vi "generateModels_v1.vi"() -> ()   [LabVIEW 2019]
panel:
  in  "DEV scan no":string="0011"
  out "SCAN_NO":string
  out "PC Processed":bool
  out "ACh Processed":bool
  in  "Build Model":bool
  in  "Process VSCAN":bool
  in  "stop":bool
  # ">>>"
  # ">>>"
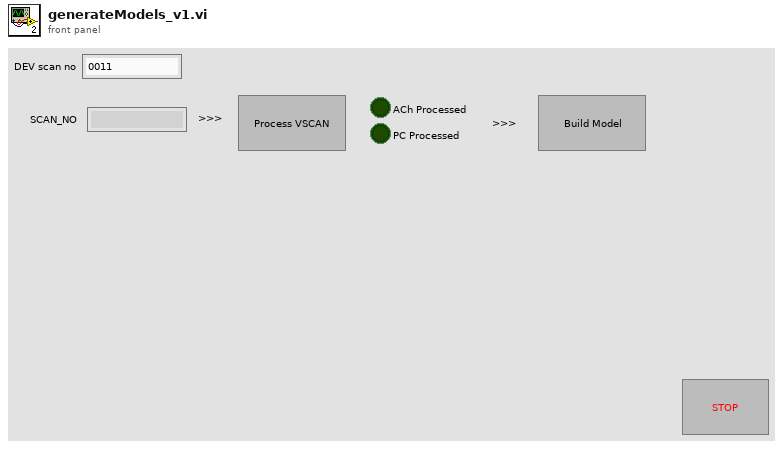
[diagram p1: front panel]
types:
  T1 = enum8{"Enabled", "Disabled", "Disabled and Grayed Out"}
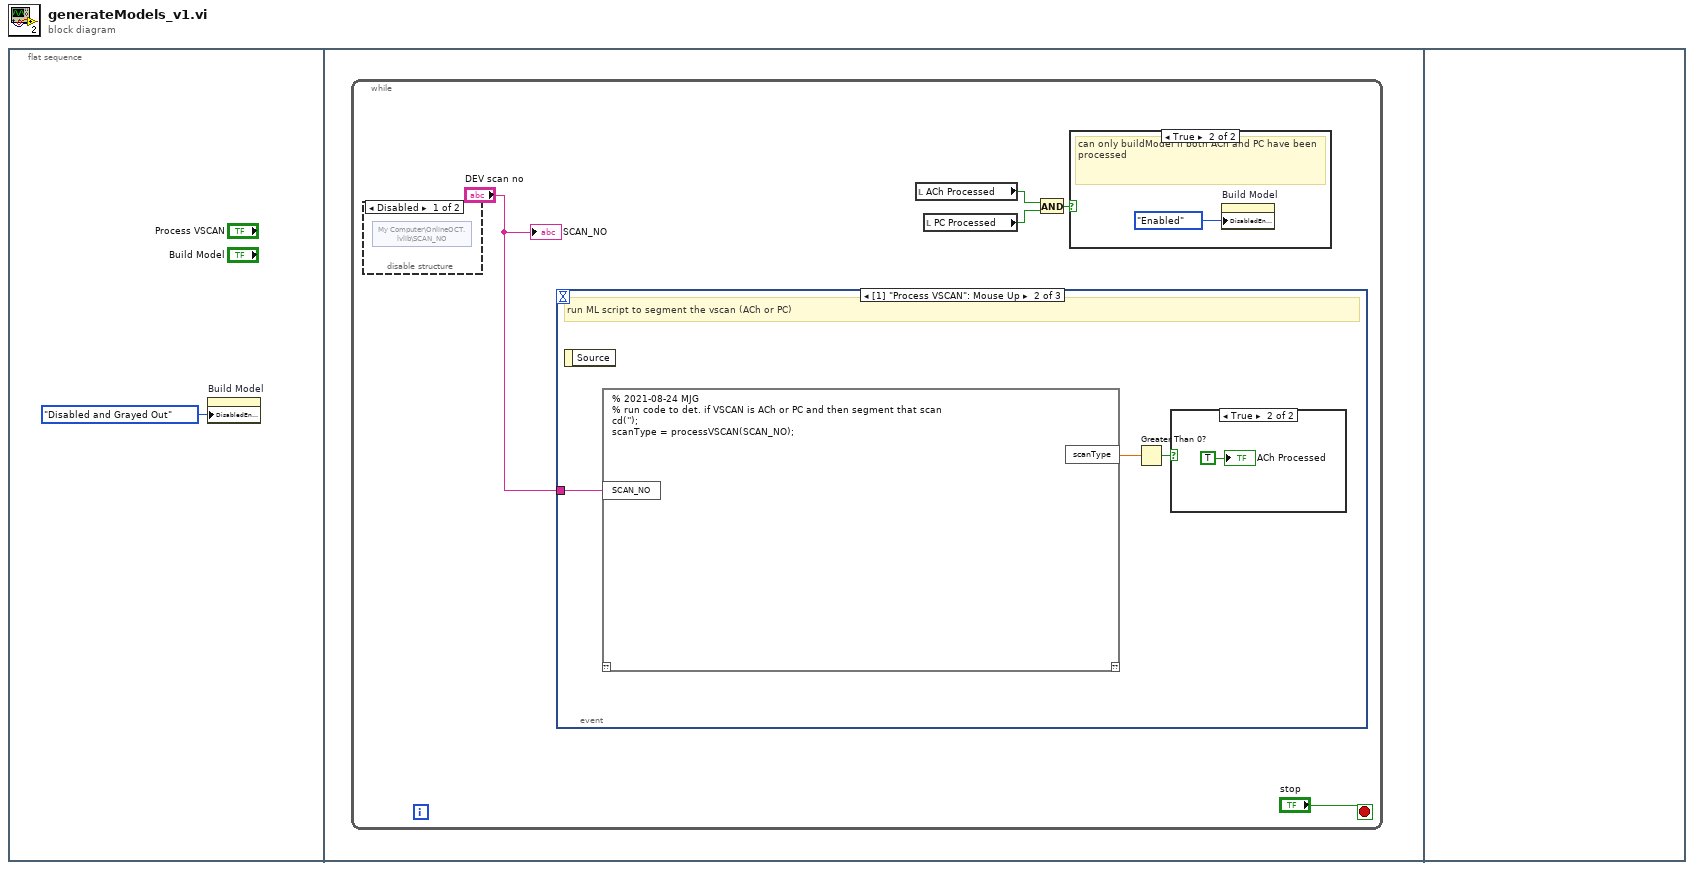
[diagram p0: block diagram]
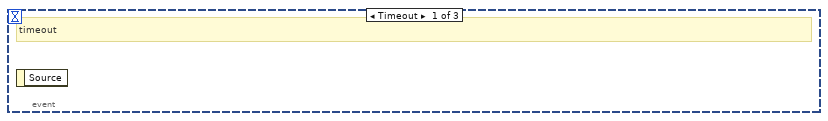
[diagram p4: hidden frame]
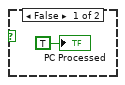
[diagram p5: hidden frame]
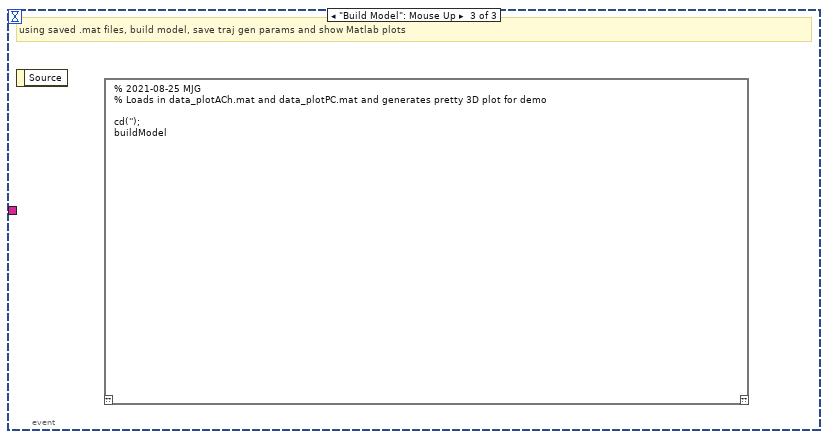
[diagram p6: hidden frame]
diagram:
  n1 = flat-sequence {
    frame #0 {
      n2 = property on="Build Model" class="Bool"("DisabledEnum"=T1."Disabled and Grayed Out" ("Disabled")) -> ()  [unwired: 2 in, 2 out]
    }
    frame #1 {
      n3 = while {
        stop <- "stop" stop-if-true
        n4 = disable-structure shown="Disabled" {
          frame Disabled {
            n5 = shared-variable "My Computer\\OnlineOCT.lvlib\\SCAN_NO"() -> ()  [unwired: 1 in, 2 out]
          }
          frame Enabled {
          }
        }
        n6 = event shown="[1] \"Process VSCAN\": Mouse Up" {
          selector: _ -> [_ _ _]
          dyn-events: _ -> [_ _ _]
          timeout: _ -> [_ _ _]
          tunnel: "DEV scan no" -> [_ w10 _]
          event Timeout {
            # "timeout"
            n7 = event-data() -> ()  [unwired: 1 in, 1 out]
          }
          event "Process VSCAN": Mouse Up {
            # "run ML script to segment the vscan (ACh or PC)"
            n8 = event-data() -> ()  [unwired: 1 in, 1 out]
            n9 = script code="% 2021-08-24 MJG \n% run code to det. if VSCAN is ACh or PC and then segment that scan\ncd('');\nscanType = processVSCAN(SCAN_NO);"("SCAN_NO"=w10) -> ("scanType"=w9:dbl)  [unwired: 1 in, 1 out]
            n10 = Greater Than 0?(x=w9) -> (x > 0?=w8:bool)
            n11 = case shown="True" w8 {
              frame False {
                "PC Processed" <- TRUE ("PC Processed")
              }
              frame True {
                "ACh Processed" <- TRUE ("ACh Processed")
              }
            }
          }
          event "Build Model": Mouse Up {
            # "using saved .mat files, build model, save traj gen params and show Matlab plots"
            n12 = event-data() -> ()  [unwired: 1 in, 1 out]
            n13 = script code="% 2021-08-25 MJG \n% Loads in data_plotACh.mat and data_plotPC.mat and generates pretty 3D plot for demo\n\ncd('');\nbuildModel"() -> ()  [unwired: 1 in, 1 out]
          }
        }
        n14 = local read "ACh Processed"() -> (w4:bool)
        n15 = local read "PC Processed"() -> (w2:bool)
        n16 = And(x=w4, y=w2) -> (x .and. y?=w3:bool)
        n17 = case shown="True" w3 {
          frame False {
          }
          frame True {
            # "can only buildModel if both ACh and PC have been processed"
            n18 = property on="Build Model" class="Bool"("DisabledEnum"=T1."Enabled" ("Disabled")) -> ()  [unwired: 2 in, 2 out]
          }
        }
        "SCAN_NO" <- "DEV scan no"
      }
    }
    frame #2 {
    }
  }
